vi "Device_List_and_Init.vi"(1 "DevInitNmb":u8) -> (0 "DevGeneralNmb":u8)   [LabVIEW 2022 SP3]
uses:
  adcDLL_0001.dll
panel:
  # "If DevInitNmb=0, shows number of spectrometers\nconnected to computer \nIf DevInitNmb!=0,  parameter does not return anything\nmeaningful"
  # "If set to 0, DevGeneralNmb will show\nnumber of spectrometers connected to \ncomputer.\nOtherwise should be set equal to the\nspectrometer number you want to initialize"
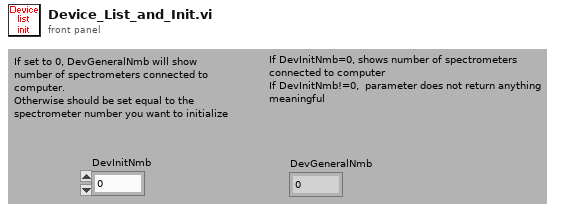
[diagram p1: front panel]
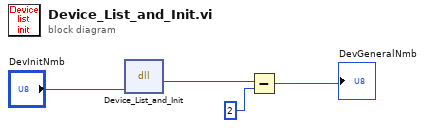
[diagram p0: block diagram]
diagram:
  n1 = dll-call lib="D:/LabVIEWSuite_64_OS/Spectrometers/ASEQ LR1/adcDLL_0001.dll" fn="Device_List_and_Init"("DevInitNmb"="DevInitNmb") -> ("return type"=w3:u8)  [unwired: 4 in, 2 out]
  n2 = Subtract(x=w3, y=u8 2) -> (x-y=→"DevGeneralNmb":u8)
